vi "SetTC0608.vi"(0 "object in":refnum<class "Application.lvclass">, 1 "TC0608":refnum<class "TC0608.lvclass">, 5 "error in (no error)":errorcluster) -> (14 "object out":refnum<class "Application.lvclass">, 19 "error out":errorcluster)   [LabVIEW 2023, in "Application.lvclass"]
uses:
  Application.lvclass
  Application.lvclass/Application.ctl
  TC0608_class/TC0608.lvclass
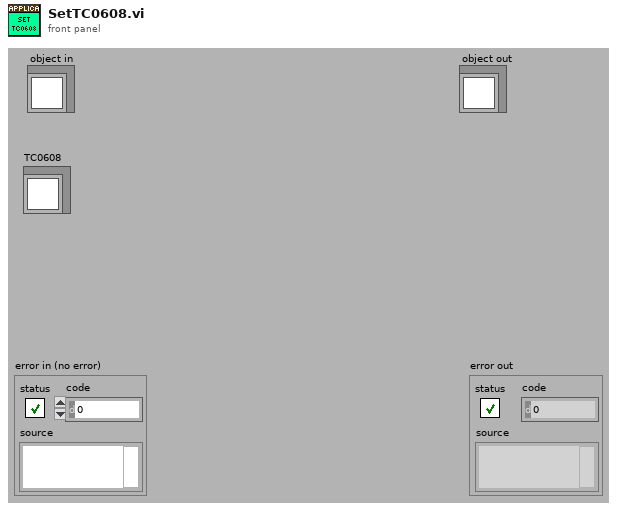
[diagram p1: front panel]
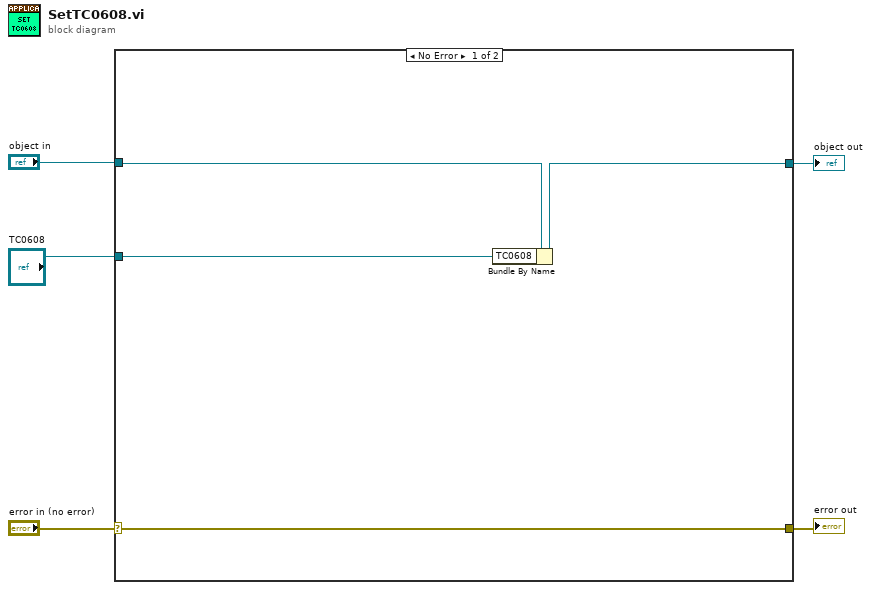
[diagram p0: block diagram]
diagram:
  n1 = case shown="No Error" "error in (no error)" {
    selector: "error in (no error)" -> [w8 w11]
    tunnel: [w8 w11] -> w4
    tunnel: [w6 w10] -> w2
    tunnel: "object in" -> [w7 w10]
    tunnel: "TC0608" -> [w9 _]
    frame No Error {
      n2 = Bundle By Name(cluster=w7, "TC0608"=w9) -> (w6:refnum<class "Application.lvclass">)
    }
    frame Error {
    }
  }
  "error out" <- w4
  "object out" <- w2
